vi "fo_MoveSCU.vi"(6 "ServerInfo":T1={"port"=104, "AEtitle"="MEDIMATIC", "host"="213.165.94.158", "remoteAE"="MEDIMATIC"}, 8 "error in (no error)":errorcluster, 9 "sopInstanceUid":string, 10 "seriesInstanceUid":string, 11 "studyInstanceUid":string) -> (0 "error out":errorcluster)   [LabVIEW 2013, in "main.lvlib"]
uses:
  main.lvlib
  C:/Users/Simon/SkyDrive/LabView/2013/DM2020/bin/Dicom.dll
  bin/Dicom.dll
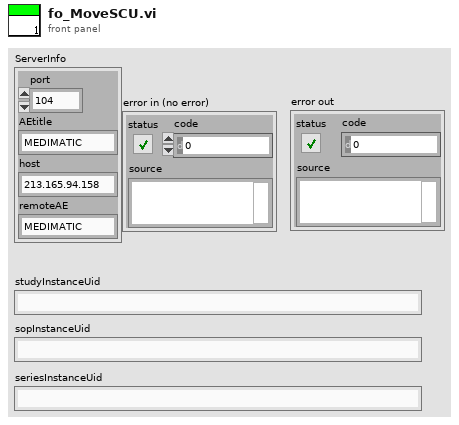
[diagram p1: front panel]
types:
  T1 = cluster{"port":i32, "AEtitle":string, "host":string, "remoteAE":string}
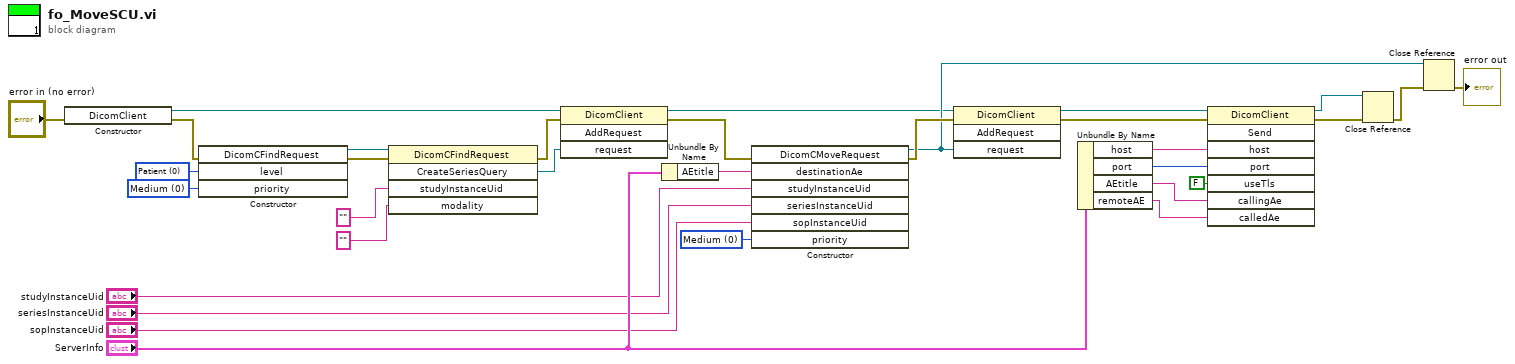
[diagram p0: block diagram]
diagram:
  w1 = u16 0 items=["Medium", "High", "Low"] ("priority")
  w13 = 0 items=["Patient", "Study", "Series", "Image", "Worklist"] ("level")
  w17 = u16 0 items=["Medium", "High", "Low"] ("priority")
  n1 = constructor class="DicomClient"(error in="error in (no error)") -> (reference out=w8:refnum<k24>, error out=w10:errorcluster)  [unwired: 2 in, 1 out]
  n2 = constructor class="DicomCFindRequest"(error in=w10, "level"=w13, "priority"=w1) -> (reference out=w12:refnum<k24>, error out=w9:errorcluster)  [unwired: 2 in, 3 out]
  n3 = invoke class="DicomCFindRequest" method="CreateSeriesQuery"(reference=w12, error in=w9, "studyInstanceUid"="" ("modality"), "modality"="") -> (error out=w7:errorcluster, "CreateSeriesQuery"=w4:refnum<k24>)  [unwired: 1 in, 3 out]
  n4 = invoke class="DicomClient" method="AddRequest"(reference=w8, error in=w7, "request"=w4) -> (reference out=w5:refnum<k24>, error out=w6:errorcluster)  [unwired: 1 in, 2 out]
  n5 = Unbundle By Name("ServerInfo") -> ("AEtitle"=w18:string)
  n6 = constructor class="DicomCMoveRequest"(error in=w6, "destinationAe"=w18, "studyInstanceUid"="studyInstanceUid", "seriesInstanceUid"="seriesInstanceUid", "sopInstanceUid"="sopInstanceUid", "priority"=w17) -> (reference out=w14:refnum<k24>, error out=w19:errorcluster)  [unwired: 2 in, 6 out]
  n7 = invoke class="DicomClient" method="AddRequest"(reference=w5, error in=w19, "request"=w14) -> (reference out=w32:refnum<k24>, error out=w24:errorcluster)  [unwired: 1 in, 2 out]
  n8 = Unbundle By Name("ServerInfo") -> ("host"=w30:string, "port"=w29:i32, "AEtitle"=w28:string, "remoteAE"=w27:string)
  n9 = invoke class="DicomClient" method="Send"(reference=w32, error in=w24, "host"=w30, "port"=w29, "useTls"=FALSE, "callingAe"=w28, "calledAe"=w27) -> (reference out=w21:refnum<k24>, error out=w23:errorcluster)  [unwired: 1 in, 6 out]
  n10 = Close Reference(reference=w21, error in (no error)=w23) -> (error out=w22:errorcluster)
  n11 = Close Reference(reference=w14, error in (no error)=w22) -> (error out=→"error out":errorcluster)
